vi "GetPDPCurrents.vi"() -> (2 "PDP Currents":dbl[](array[numeric]))   [LabVIEW 2017]
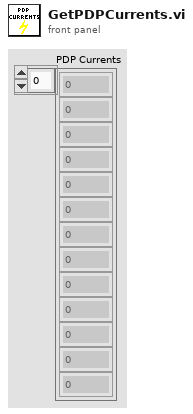
[diagram p1: front panel]
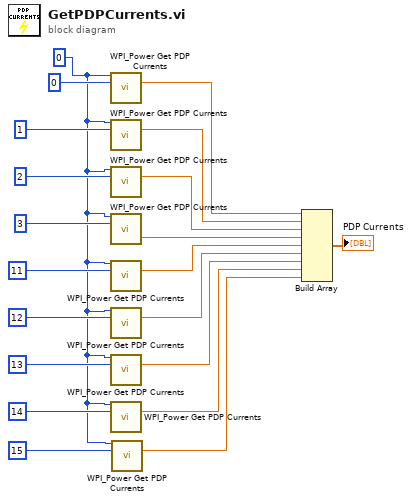
[diagram p0: block diagram]
diagram:
  w1 = 0 ("PDP Channel")
  n1 = call <vilib>:"WPI_Power Get PDP Currents.vi"("Power Distribution Panel (0)"=w1, "PDP Channel"=0) -> ("current (A)"=w13:dbl)  [unwired: 11 in, 2 out]
  n2 = call <vilib>:"WPI_Power Get PDP Currents.vi"("Power Distribution Panel (0)"=w1, "PDP Channel"=1) -> ("current (A)"=w12:dbl)  [unwired: 11 in, 2 out]
  n3 = call <vilib>:"WPI_Power Get PDP Currents.vi"("Power Distribution Panel (0)"=w1, "PDP Channel"=2) -> ("current (A)"=w11:dbl)  [unwired: 11 in, 2 out]
  n4 = call <vilib>:"WPI_Power Get PDP Currents.vi"("Power Distribution Panel (0)"=w1, "PDP Channel"=3) -> ("current (A)"=w10:dbl)  [unwired: 11 in, 2 out]
  n5 = call <vilib>:"WPI_Power Get PDP Currents.vi"("Power Distribution Panel (0)"=w1, "PDP Channel"=11) -> ("current (A)"=w9:dbl)  [unwired: 11 in, 2 out]
  n6 = call <vilib>:"WPI_Power Get PDP Currents.vi"("Power Distribution Panel (0)"=w1, "PDP Channel"=12) -> ("current (A)"=w8:dbl)  [unwired: 11 in, 2 out]
  n7 = call <vilib>:"WPI_Power Get PDP Currents.vi"("Power Distribution Panel (0)"=w1, "PDP Channel"=13) -> ("current (A)"=w7:dbl)  [unwired: 11 in, 2 out]
  n8 = call <vilib>:"WPI_Power Get PDP Currents.vi"("Power Distribution Panel (0)"=w1, "PDP Channel"=14) -> ("current (A)"=w6:dbl)  [unwired: 11 in, 2 out]
  n9 = call <vilib>:"WPI_Power Get PDP Currents.vi"("Power Distribution Panel (0)"=w1, "PDP Channel"=u8 15 ("PDP (0)")) -> ("current (A)"=w3:dbl)  [unwired: 11 in, 2 out]
  n10 = Build Array(w13, w12, w11, w10, w9, w8, w7, w6, w3) -> (→"PDP Currents":dbl[])
